vi "Пылесос.vi"() -> ()   [LabVIEW 2021]
uses:
  Up1.ctl
  Left1.ctl
  Right1.ctl
panel:
  out "Down":bool
  out "Right":T1
  in  "Left":T2
  in  "Up":T3
  out "Пылесос":bool
  out "Заряд":u8(slide) scale=0.0..100.0
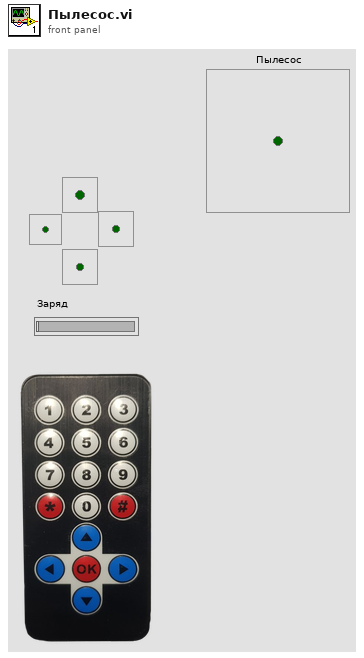
[diagram p1: front panel]
types:
  T1 = typedef "Right1.ctl" = bool
  T2 = typedef "Left1.ctl" = bool
  T3 = typedef "Up1.ctl" = bool
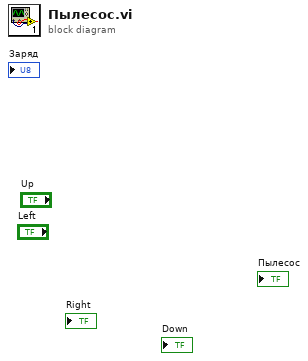
[diagram p0: block diagram]
diagram:
